vi "CODE_WRITE_PORT.vi"(11 "Array":bool[](array[boolean])) -> (3 "number":u16)   [LabVIEW 2019]
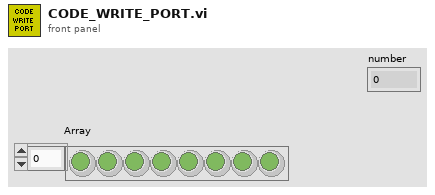
[diagram p1: front panel]
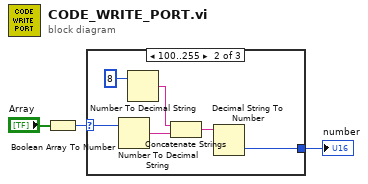
[diagram p0: block diagram]
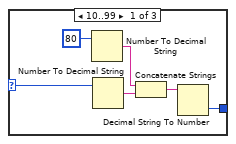
[diagram p2: hidden frame]
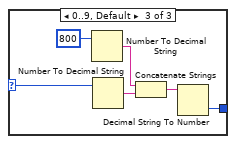
[diagram p3: hidden frame]
diagram:
  n1 = Boolean Array To Number(Boolean array="Array") -> (number=w2:u32)
  n2 = case shown="100..255" w2 {
    selector: w2 -> [w5 w11 w20]
    tunnel: [w4 w10 w16] -> w1
    frame 10..99 {
      n3 = Number To Decimal String(number=80) -> (decimal integer string=w8:string)  [unwired: 1 in]
      n4 = Number To Decimal String(number=w5) -> (decimal integer string=w7:string)  [unwired: 1 in]
      n5 = Concatenate Strings(w8, w7) -> (w6:string)
      n6 = Decimal String To Number(string=w6) -> (number=w4:i32)  [unwired: 2 in, 1 out]
    }
    frame 100..255 {
      n7 = Number To Decimal String(number=w11) -> (decimal integer string=w13:string)  [unwired: 1 in]
      n8 = Number To Decimal String(number=8) -> (decimal integer string=w14:string)  [unwired: 1 in]
      n9 = Concatenate Strings(w14, w13) -> (w12:string)
      n10 = Decimal String To Number(string=w12) -> (number=w10:i32)  [unwired: 2 in, 1 out]
    }
    frame 0..9, Default {
      n11 = Number To Decimal String(number=800) -> (decimal integer string=w19:string)  [unwired: 1 in]
      n12 = Number To Decimal String(number=w20) -> (decimal integer string=w18:string)  [unwired: 1 in]
      n13 = Concatenate Strings(w19, w18) -> (w17:string)
      n14 = Decimal String To Number(string=w17) -> (number=w16:i32)  [unwired: 2 in, 1 out]
    }
  }
  "number" <- w1
